vi "Create TDMS Channels.vi"(5 "XNET Cluster":refnum<k21>="ManyXnetChannels", 7 "CAN Interface":refnum<k21>="CAN1", 8 "error in (no error)":errorcluster, 10 "group name in":string="Log", 11 "TDMS ref in":refnum<k34>) -> (0 "error out":errorcluster, 1 "Signal Names":string[](array[string]), 2 "group name out":string="Log", 3 "TDMS ref out":refnum<k34>, 4 "Signal Units":string[](array[string]))   [LabVIEW 2021, in "XNET-CAN-Signal-Logger.lvlib"]
uses:
  XNET-CAN-Signal-Logger.lvlib
  <resource>/objmgr/xnet.rc
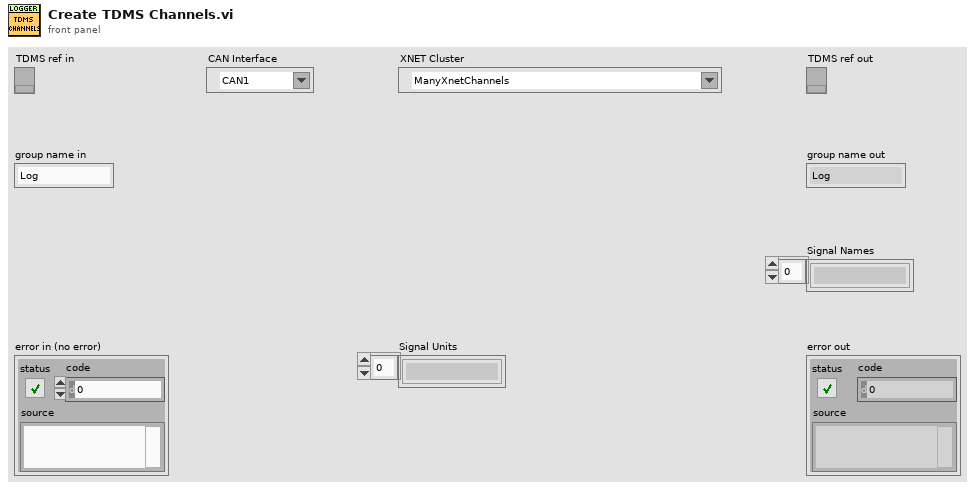
[diagram p1: front panel]
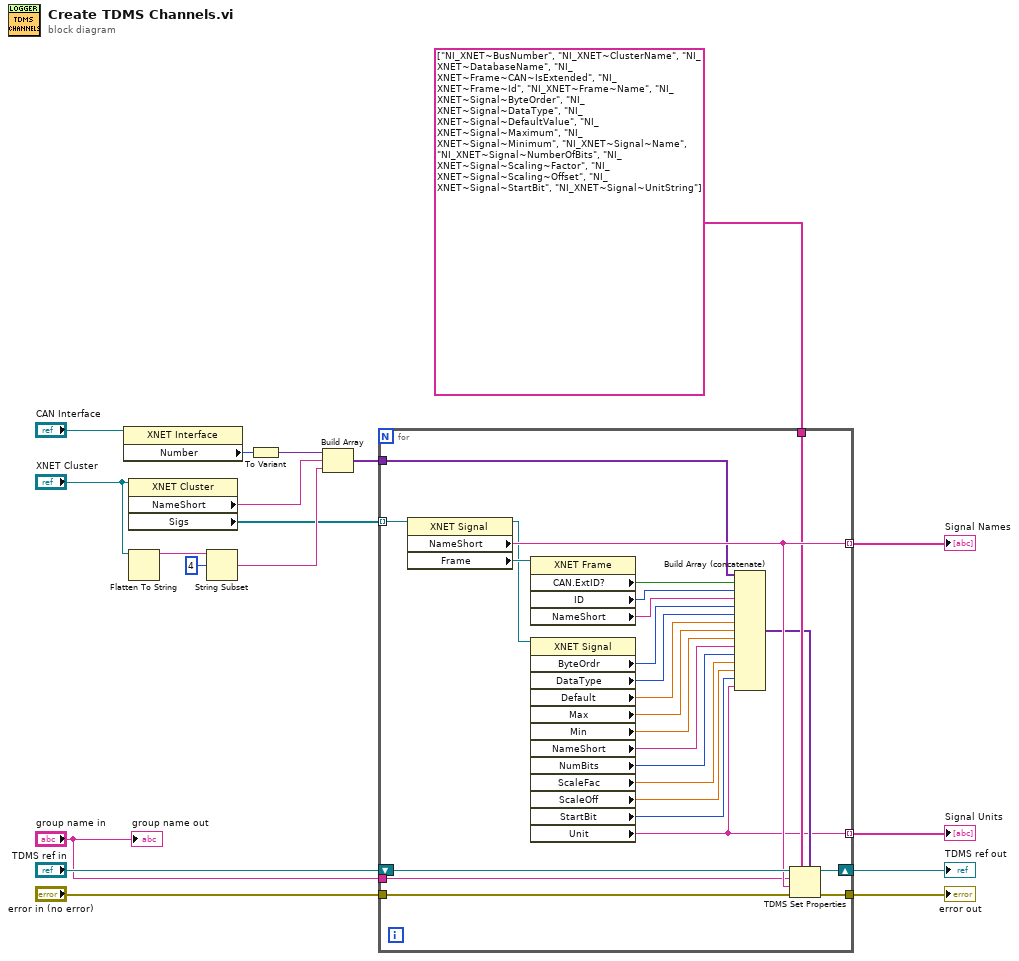
[diagram p0: block diagram]
diagram:
  n1 = property class="XNET Interface"(reference="CAN Interface") -> ("Number"=w9:u32)  [unwired: 1 in, 2 out]
  n2 = property class="XNET Cluster"(reference="XNET Cluster") -> ("NameShort"=w2:string, "Sigs"=w6:refnum<k21>[])  [unwired: 1 in, 2 out]
  n3 = Flatten To String(anything="XNET Cluster") -> (data string=w11:string)  [unwired: 3 in, 2 out]
  n4 = String Subset(string=w11, offset (0)=4) -> (substring=w7:string)  [unwired: 1 in]
  n5 = To Variant(anything=w9) -> (Variant=w8:variant)
  n6 = Build Array(w8, w2, w7) -> (w5:variant[])
  n7 = for {
    tunnel: w6 -> [w44] mode=indexing
    tunnel: [w42] -> w14 mode=indexing
    shift-right: [w40] -> w16
    shift-left: "TDMS ref in" -> [w43]
    tunnel: "error in (no error)" -> [w41]
    tunnel: [w39] -> w18
    tunnel: string[] ["NI_XNET~BusNumber", "NI_XNET~ClusterName", "NI_XNET~DatabaseName", "NI_XNET~Frame~CAN~IsExtended", "NI_XNET~Frame~Id", "NI_XNET~Frame~Name", "NI_XNET~Signal~ByteOrder", "NI_XNET~Signal~DataType", "NI_XNET~Signal~DefaultValue", "NI_XNET~Signal~Maximum", "NI_XNET~Signal~Minimum", "NI_XNET~Signal~Name", "NI_XNET~Signal~NumberOfBits", "NI_XNET~Signal~Scaling~Factor", "NI_XNET~Signal~Scaling~Offset", "NI_XNET~Signal~StartBit", "NI_XNET~Signal~UnitString"] ("property names") -> [w38]
    tunnel: w5 -> [w35]
    tunnel: "group name in" -> [w20]
    tunnel: [w19] -> w3 mode=indexing
    n8 = property class="XNET Signal"(reference=w44) -> (reference out=w36:refnum<k21>, "NameShort"=w42:string, "Frame"=w37:refnum<k21>)  [unwired: 1 in, 1 out]
    n9 = property class="XNET Frame"(reference=w37) -> ("CAN.ExtID?"=w33:bool, "ID"=w32:u32, "NameShort"=w31:string)  [unwired: 1 in, 2 out]
    n10 = property class="XNET Signal"(reference=w36) -> ("ByteOrdr"=w30:u32, "DataType"=w29:u32, "Default"=w28:dbl, "Max"=w27:dbl, "Min"=w26:dbl, "NameShort"=w25:string, "NumBits"=w24:u32, "ScaleFac"=w23:dbl, "ScaleOff"=w22:dbl, "StartBit"=w21:u32, "Unit"=w19:string)  [unwired: 1 in, 2 out]
    n11 = Build Array (concatenate)(w35, w33, w32, w31, w30, w29, w28, w27, w26, w25, w24, w23, w22, w21, w19) -> (w34:variant[])
    n12 = TDMS Set Properties(5:w34, 7:w38, 8:w41, 9:w42, 10:w20, 11:w43) -> (0:w39:errorcluster, 3:w40:refnum<k34>)  [unwired: 2 out]
  }
  "error out" <- w18
  "TDMS ref out" <- w16
  "Signal Names" <- w14
  "Signal Units" <- w3
  "group name out" <- "group name in"
